vi "UI_Unit_Start.vi"() -> ()   [LabVIEW 2014]
panel:
  out "时间倒计时：":string
  in  "齿轮箱油站当前状态":i32(listbox) caption="当前状态"
  in  "试验当前状态":i32(listbox) caption="当前状态"
  in  "陪试当前状态 2":i32(listbox) caption="当前状态"
  in  "比例加载系统当前状态":i32(listbox) caption="当前状态"
  out "6220轴向液压缸加载压力":dbl caption="轴向液压缸加载压力"
  out "6220径向液压缸加载压力":dbl caption="径向液压缸加载压力"
  out "油站系统综合状态异常":bool
  in  "供油流量异常":bool
  in  "供油压力异常":bool
  in  "齿轮子系统2号油泵故障":bool caption="2号油泵故障"
  in  "齿轮子系统1号油泵故障":bool caption="1号油泵故障"
  in  "回油泵故障":bool
  in  "齿轮子系统循散热器风机故障":bool caption="散热器风机故障"
  in  "齿轮子系统供油过滤器压差过高":bool caption="供油过滤器压差过高"
  in  "齿轮子系统油箱液位过低":bool caption="油箱液位过低"
  in  "齿轮子系统油箱液位过高":bool caption="油箱液位过高"
  in  "齿轮子系统加热装置异常":bool caption="油箱加热器异常"
  out "齿轮箱油站供油压力":dbl caption="供油压力"
  out "齿轮箱轴承温度":dbl
  out "齿轮箱油站供油油温":dbl caption="供油油温"
  out "油箱1油液温度":dbl caption="油箱温度"
  out "油站系统综合状态":bool
  out "过滤器压差":bool
  out "供油流量状态":bool
  out "散热器风机状态":bool
  out "回油泵状态":bool
  out "2号油泵状态":bool
  out "1号油泵状态":bool
  out "油箱润滑油液位":bool
  out "陪试回油滤油发讯":bool caption="油箱温度发讯"
  out "陪试吸油滤油发讯":bool caption="吸油滤油发讯"
  out "陪试回油滤油发讯":bool caption="回路滤油发讯"
  out "陪试回油滤油发讯":bool caption="回油滤油发讯"
  out "陪试管路滤油发讯":bool caption="管路滤油发讯"
  out "油箱液位低":bool
  out "油箱液位高":bool
  out "陪试供油流量":dbl caption="供油流量"
  out "陪试高低压供油选择":dbl caption="高低压供油选择"
  out "副油箱温度发讯":bool
  out "主油箱温度发讯":bool
  out "吸油滤油发讯":bool
  out "回油滤油发讯":bool
  out "管路滤油发讯":bool
  out "回路滤油发讯":bool
  out "副油箱液位低":bool
  out "副油箱液位高":bool
  out "主油箱液位低":bool
  out "主油箱液位高":bool
  out "试验供油温度设定":dbl caption="供油温度"
  out "比例加载回油滤油发讯":bool
  out "比例加载高压滤油发讯":bool
  out "比例加载油箱液位低":bool
  out "比例加载油箱液位高":bool
  out "预载荷轴向液压缸加载压力":dbl caption="轴向液压缸加载压力"
  out "预载荷径向液压缸加载压力":dbl caption="径向液压缸加载压力"
  out "试验供油流量":dbl caption="供油流量"
  out "试验供油温度":dbl caption="供油温度"
  out "试验供油压力":dbl caption="供油压力"
  out "陪试供油温度":dbl caption="供油温度"
  out "陪试供油压力":dbl caption="供油压力"
  out "轴向液压缸加载压力":dbl
  out "径向液压缸加载压力":dbl
  # "单元子系统启动"
  # "比例加载系统启动"
  # "陪试轴承润滑单元启动"
  # "试验轴承润滑单元启动"
  # "齿轮箱油站启动"
  # "设置量"
  # "设置量"
  # "监测量"
  # "设置量"
  # "监测量"
  # "监测量"
  # "监测量"
  # "单元系统"
  # "传感器"
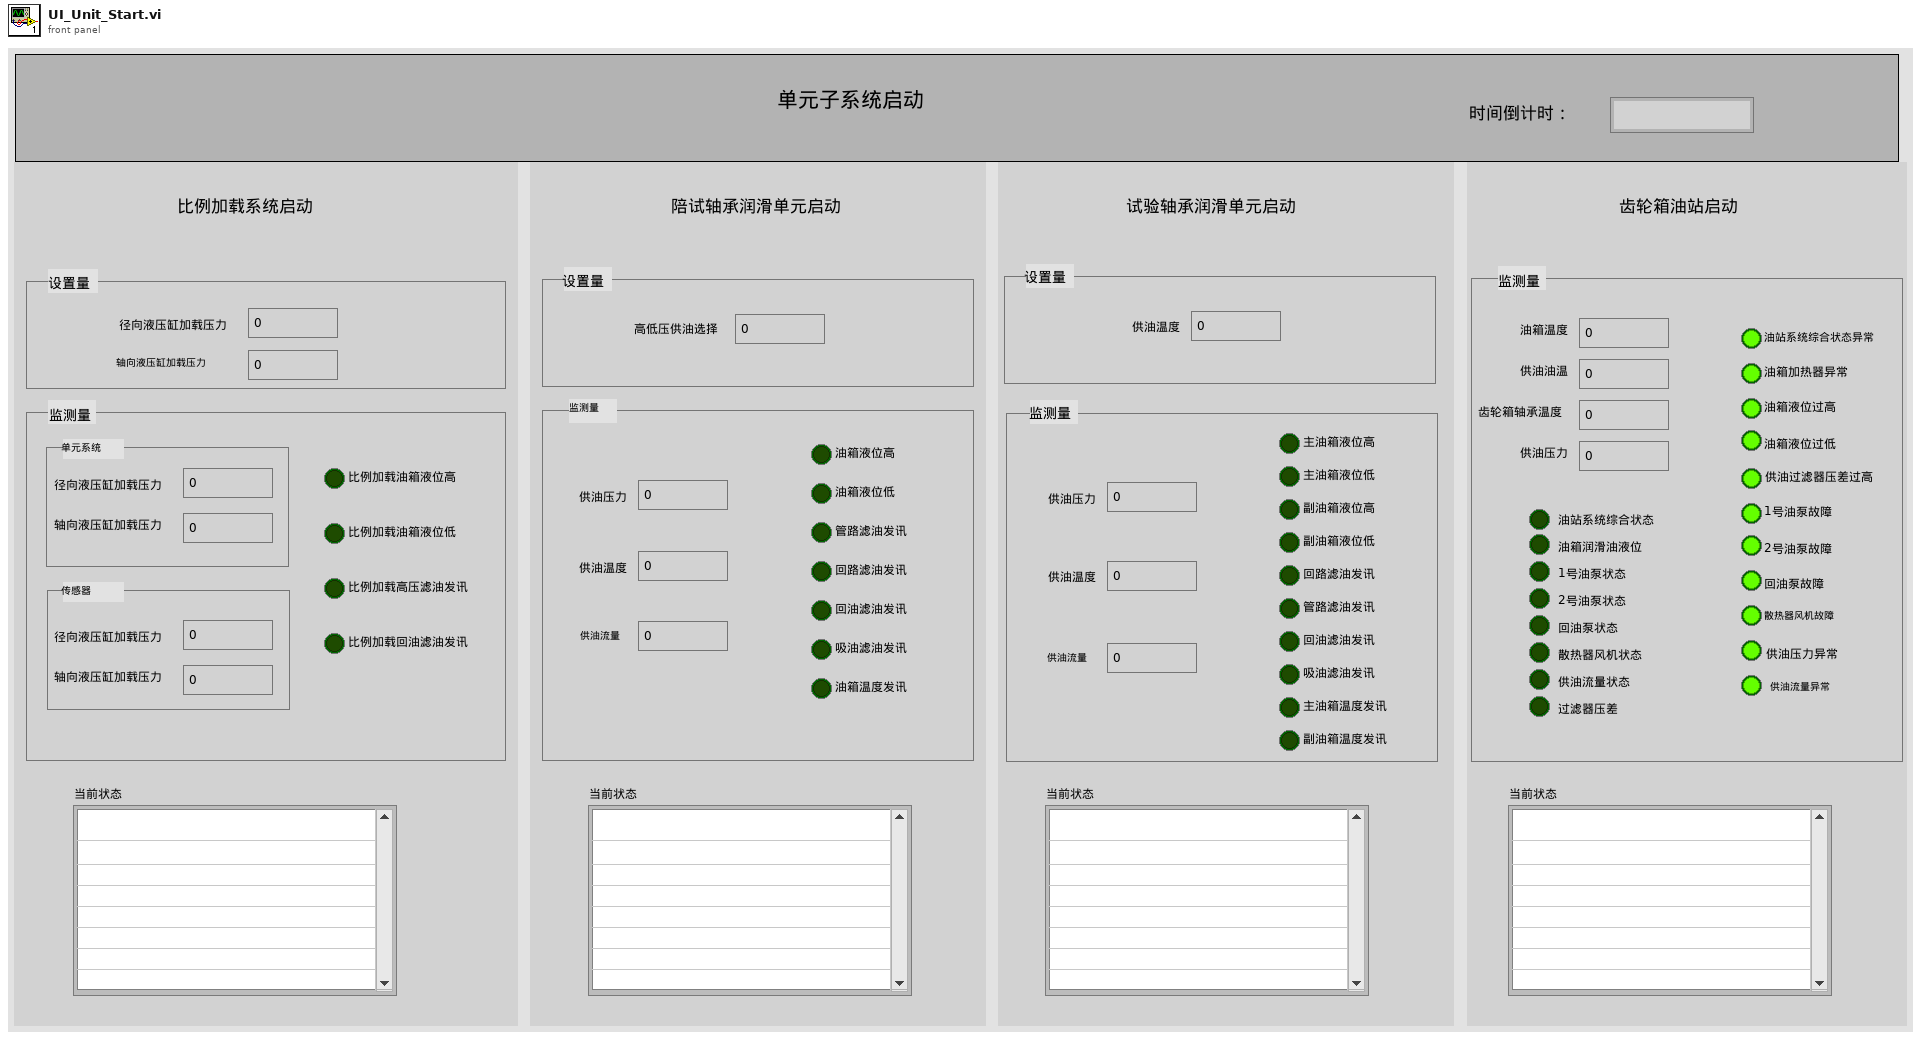
[diagram p1: front panel]
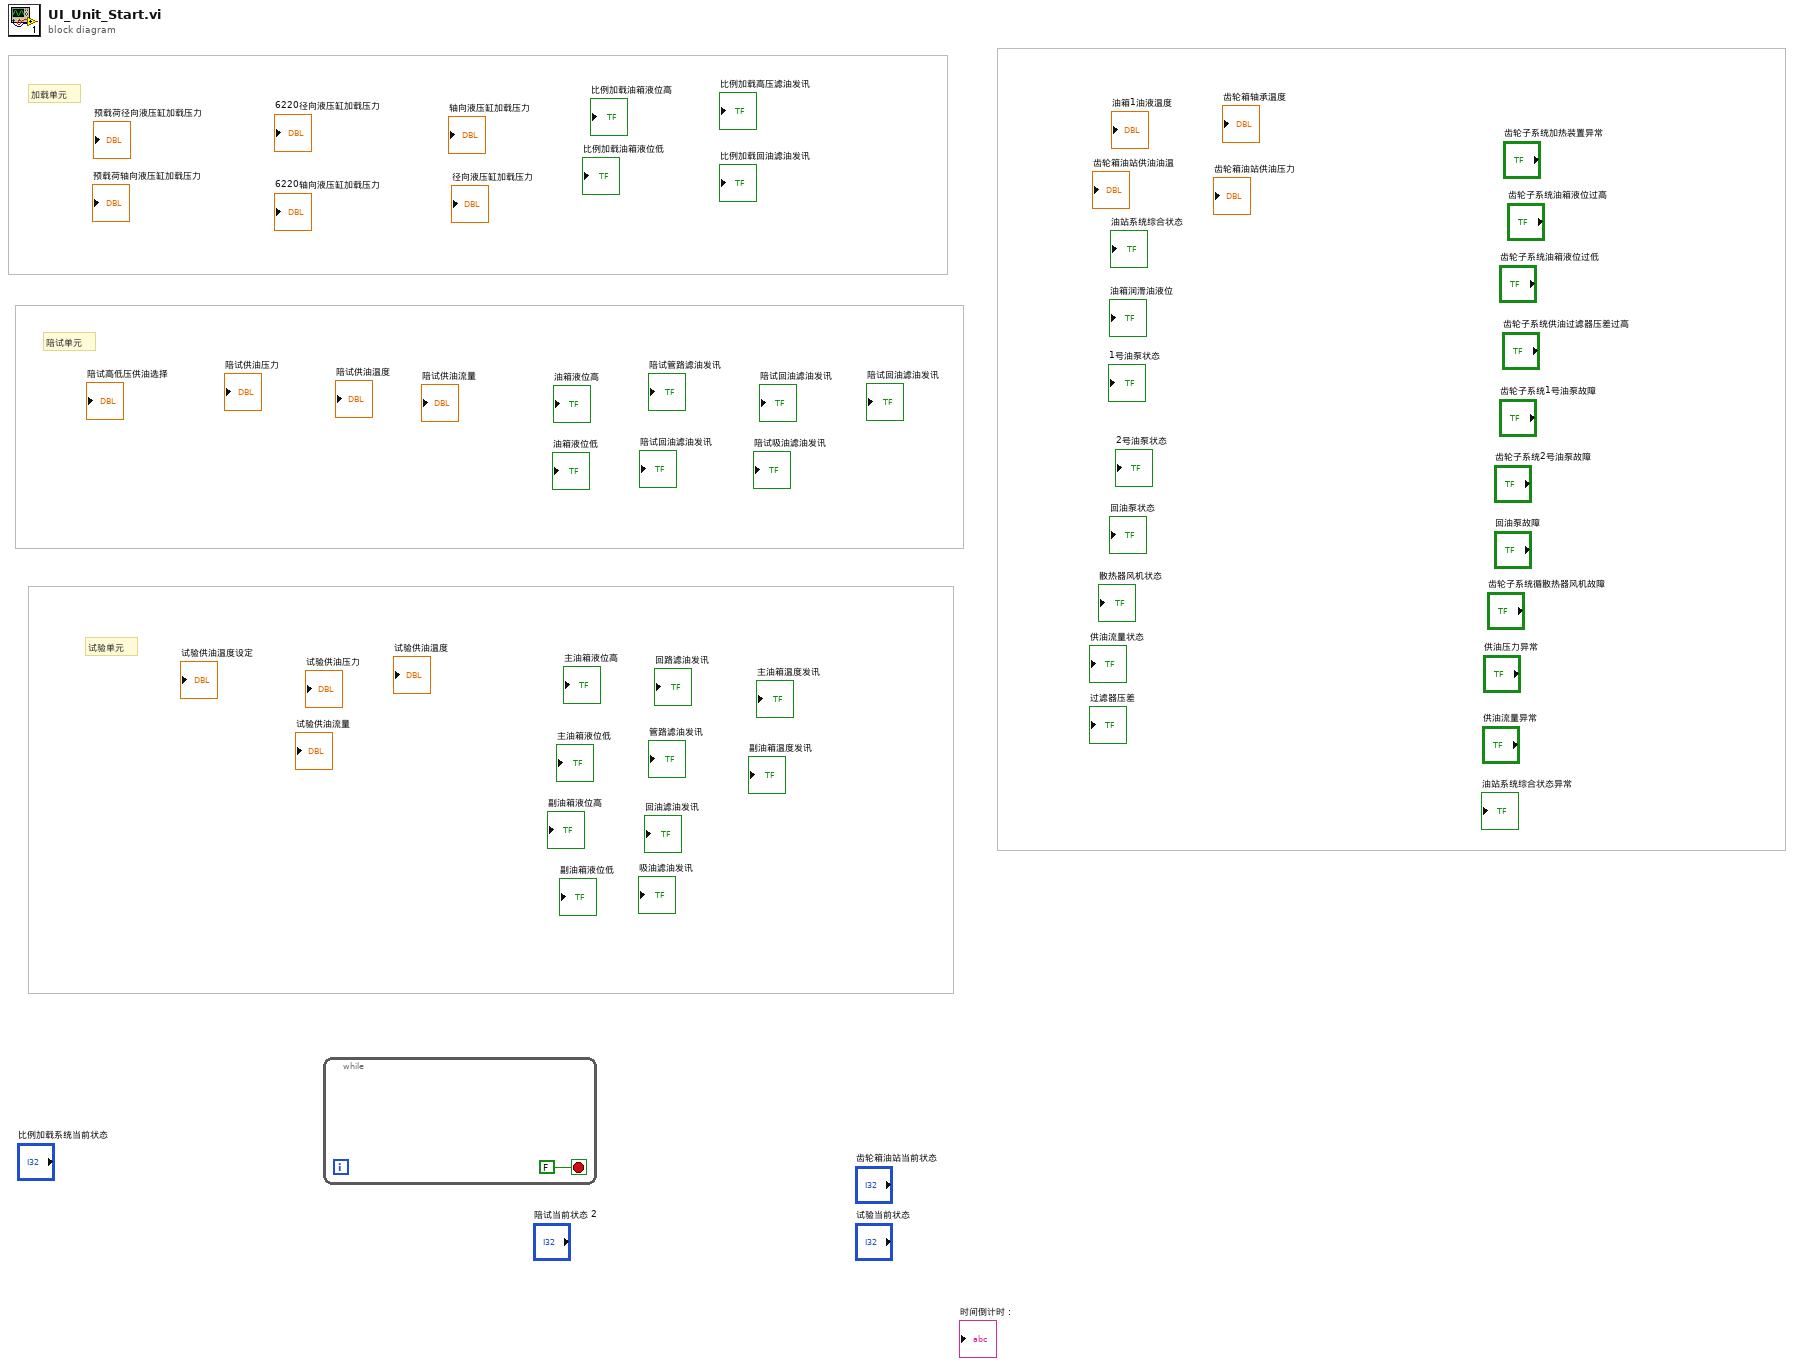
[diagram p0: block diagram]
diagram:
  # "试验单元"
  # "陪试单元"
  # "加载单元"
  n1 = while {
    stop <- FALSE stop-if-true
  }
